vi "TablaArray.vi"() -> ()   [LabVIEW 2020]
panel:
  in  "Renglones":i32
  in  "Columnas":i32
  out "Array":i32[][](array[numeric])
  out "element":i32
  in  "Columna Buscador":i32
  in  "Renglon Buscador":i32
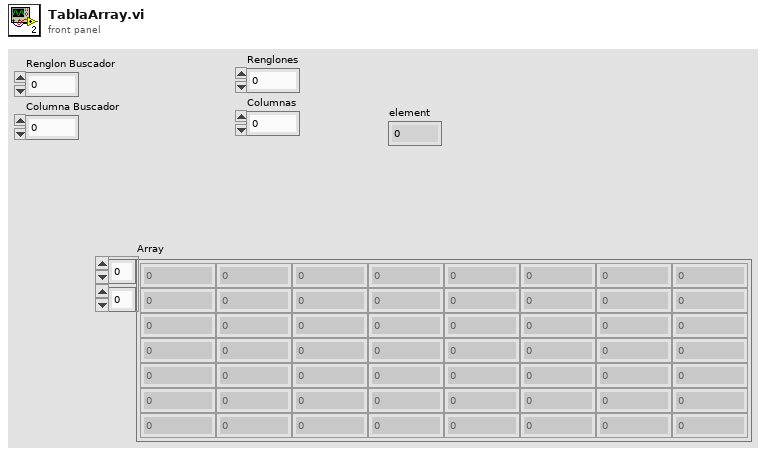
[diagram p1: front panel]
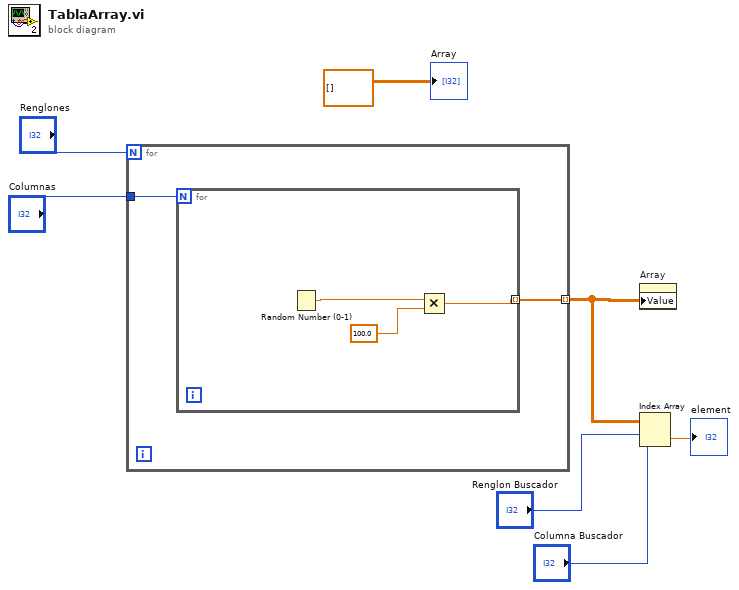
[diagram p0: block diagram]
diagram:
  n1 = for {
    N: "Renglones" -> [_]
    tunnel: "Columnas" -> [w9]
    tunnel: [w8] -> w6 mode=indexing
    n2 = for {
      N: w9 -> [_]
      tunnel: [w10] -> w8 mode=indexing
      n3 = Random Number (0-1)() -> (number: 0 to 1=w11:dbl)
      n4 = Multiply(x=w11, y=100.0) -> (x*y=w10:dbl)
    }
  }
  n5 = property on="Array" class="Arr (strict)"("Value"=w6) -> ()  [unwired: 2 in, 2 out]
  n6 = Index Array(array=w6, index (row)="Renglon Buscador", index (col)="Columna Buscador") -> (element=→"element":dbl)
  "Array" <- dbl[][] [] ("Array")
